vi "getQwgtFromFile.vi"(8 "error in (no error)":errorcluster, 11 "OptCtrl in":refnum<class "OptCtrl.lvclass">) -> (0 "error out":errorcluster, 2 "Wgt of Q":dbl[](array[numeric]), 3 "OptCtrl out":refnum<class "OptCtrl.lvclass">)   [LabVIEW 2016, in "OptCtrl.lvclass"]
doc: "Get the weighting ratio of image quality from file. This is used in the Q matrix calculation."
uses:
  OptCtrl.lvclass
  OptCtrl.lvclass/OptCtrl.ctl
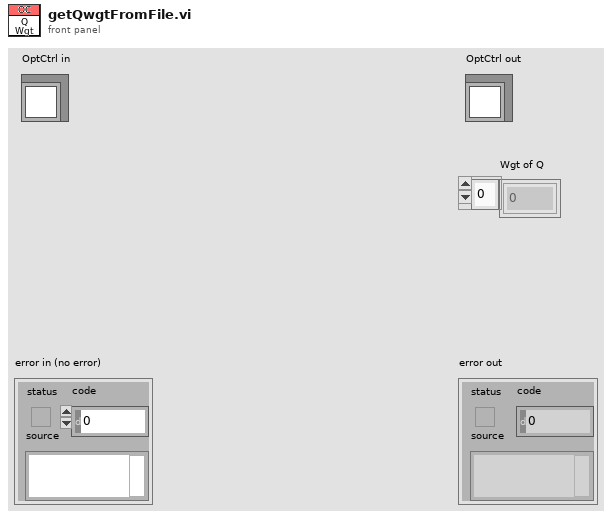
[diagram p1: front panel]
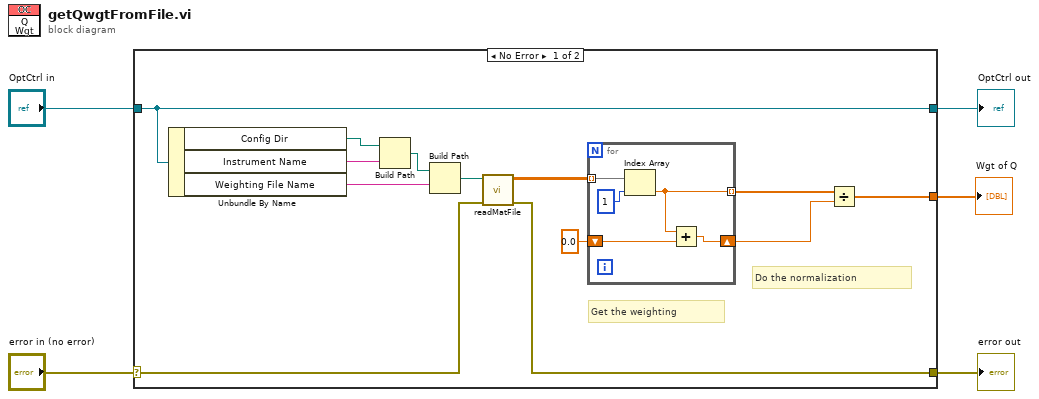
[diagram p0: block diagram]
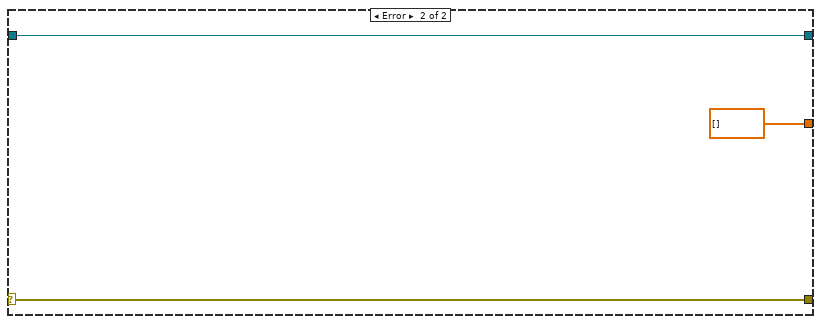
[diagram p2: hidden frame]
diagram:
  n1 = case shown="No Error" "error in (no error)" {
    selector: "error in (no error)" -> [w13 w26]
    tunnel: [w12 w26] -> w4
    tunnel: [w18 w25] -> w2
    tunnel: "OptCtrl in" -> [w18 w25]
    tunnel: [w7 dbl[] []] -> w1
    frame No Error {
      # "Do the normalization"
      # "Get the weighting"
      n2 = Unbundle By Name(w18) -> ("Config Dir"=w17:path, "Instrument Name"=w16:string, "Weighting File Name"=w6:string)
      n3 = Build Path(base path=w17, name or relative path=w16) -> (appended path=w15:path)
      n4 = Build Path(base path=w15, name or relative path=w6) -> (appended path=w14:path)
      n5 = call "readMatFile.vi"("error in (no error)"=w13, "Path"=w14) -> ("error out"=w12:errorcluster, "Matrix"=w11:dbl[][])  [unwired: 8 in]
      n6 = for {
        tunnel: w11 -> [w23] mode=indexing
        tunnel: [w21] -> w9 mode=indexing
        shift-right: [w19] -> w8
        shift-left: 0.0 -> [w20]
        n7 = Index Array(array=w23, index=1) -> (element=w21:dbl)
        n8 = Add(x=w21, y=w20) -> (x+y=w19:dbl)
      }
      n9 = Divide(x=w9, y=w8) -> (x/y=w7:dbl[])
    }
    frame Error {
    }
  }
  "error out" <- w4
  "OptCtrl out" <- w2
  "Wgt of Q" <- w1
